vi "Open.vi"(8 "Error In":errorcluster, 11 "EZ430-Chronos Config":T2) -> (0 "Error Out":errorcluster, 3 "EZ430-Chronos Ref":T1)   [LabVIEW 2011, in "LVH-EZ430.lvlib"]
uses:
  <vilib>/LabVIEW Hacker/LabVIEW Interface for EZ430-Chronos/LVH-EZ430.lvlib
  <vilib>/LabVIEW Hacker/LabVIEW Interface for EZ430-Chronos/Private/Type Defs/EZ430-Chronos Config.ctl
  <vilib>/LabVIEW Hacker/LabVIEW Interface for EZ430-Chronos/Private/Type Defs/EZ430-Chronos Ref.ctl
  <vilib>/Instr/_visa.llb/VISA Configure Serial Port (Instr).vi
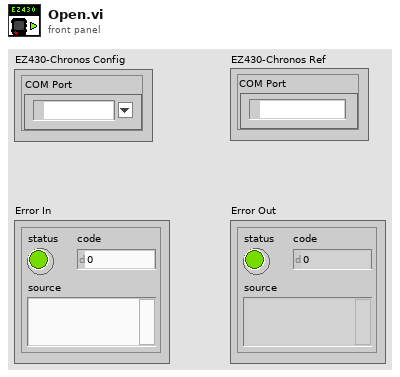
[diagram p1: front panel]
types:
  T1 = typedef "LVH-EZ430.lvlib/EZ430-Chronos Ref.ctl" = cluster{"COM Port":refnum<visa-resource-name>}
  T2 = typedef "LVH-EZ430.lvlib/EZ430-Chronos Config.ctl" = cluster{"COM Port":refnum<visa-resource-name>}
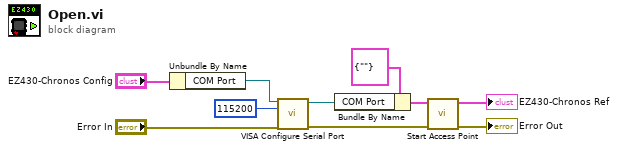
[diagram p0: block diagram]
diagram:
  n1 = Unbundle By Name("EZ430-Chronos Config") -> ("COM Port"=w9:refnum<visa-resource-name>)
  n2 = call-poly "VISA Configure Serial Port"("VISA resource name"=w9, "baud rate (9600)"=u32 115200, "error in (no error)"="Error In") -> ("VISA resource name out"=w5:refnum<visa-resource-name>, "error out"=w1:errorcluster)  [unwired: 11 in]
  n3 = Bundle By Name(cluster=T1 {"COM Port"=""} ("EZ430-Chronos Config"), "COM Port"=w5) -> (w4:T1)
  n4 = call <vilib>:"Start Access Point.vi"("Error In"=w1, "EZ430-Chronos Ref"=w4) -> ("Error Out"=→"Error Out":errorcluster, "EZ430-Chronos Ref"=→"EZ430-Chronos Ref":T1)  [unwired: 7 in, 1 out]
